vi "Build Report String.vi"(8 "error in (no error)":errorcluster, 10 "Result":T1, 11 "Timing Action in":refnum<class "Timing Action.lvclass">) -> (0 "error out":errorcluster, 2 "Report String":string, 3 "Timing Action out":refnum<class "Timing Action.lvclass">)   [LabVIEW 2020, in "MacroAssert.lvlib" / "Timing Action.lvclass"]
doc: "Builds a string using <B>Step</B> and <B>Result</B> to be included in a report."
uses:
  Timing Action.lvclass
  Timing Action.lvclass/Timing Action.ctl
  MacroAssert.lvlib
  Action Step/Action Step.lvclass
  CTLs/Result.ctl
  CTLs/Outcome.ctl
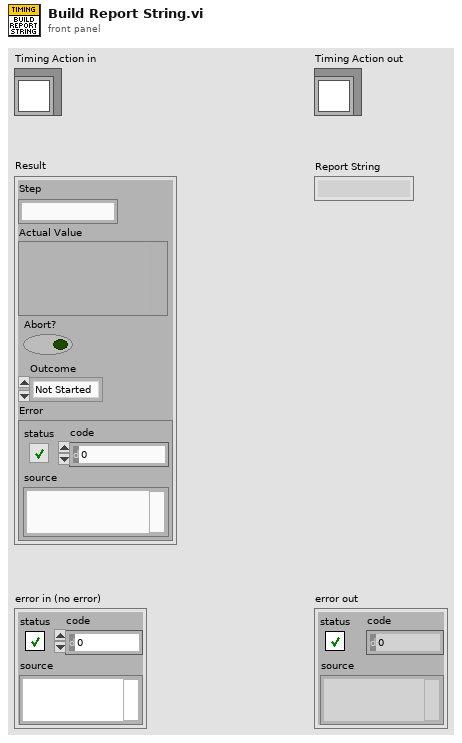
[diagram p1: front panel]
types:
  T1 = typedef "MacroAssert.lvlib/Result.ctl" = cluster{"Step":string, "Actual Value":variant, "Abort?":bool, "Outcome":T2, "Error":errorcluster}
  T2 = typedef "MacroAssert.lvlib/Outcome.ctl" = enum16{"Not Started", "Skipped", "Pass", "Fail", "Complete", "Error", "Auto Abort", "User Abort"}
  T3 = typedef "MacroAssert.lvlib/Timing Action.lvclass/Timing Action Type.ctl" = enum16{"Wait", "Wait Until"}
  T4 = typedef "MacroAssert.lvlib/Timing Action.lvclass/Time Unit.ctl" = enum16{"milliseconds", "seconds", "minutes"}
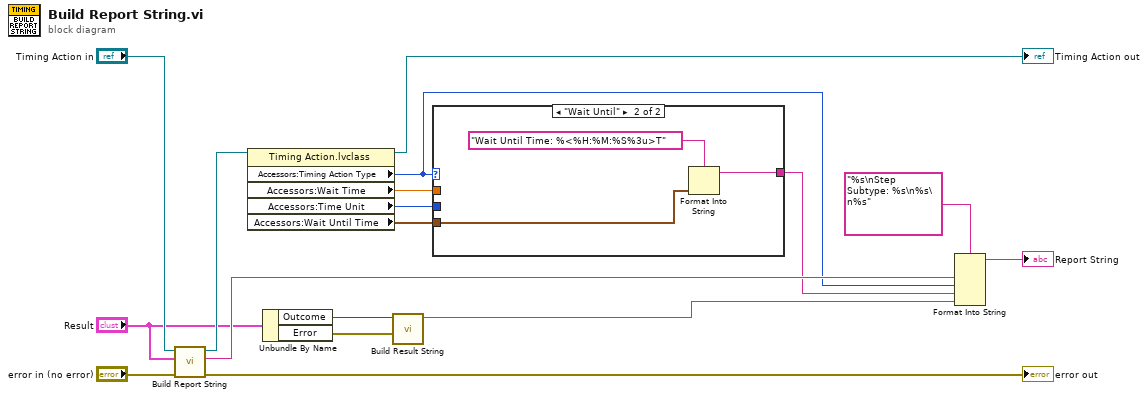
[diagram p0: block diagram]
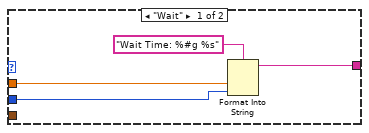
[diagram p2: hidden frame]
diagram:
  n1 = call-parent "Build Report String.vi"("error in (no error)"="error in (no error)", "Result"="Result", "Step in"="Timing Action in") -> ("error out"=→"error out":errorcluster, "Report String"=w12:string, "Step out"=w13:refnum<class "Timing Action.lvclass">)  [unwired: 6 in]
  n2 = property class="Timing Action.lvclass"(reference=w13) -> (reference out=→"Timing Action out":refnum<class "Timing Action.lvclass">, "Accessors:Timing Action Type"=w1:T3, "Accessors:Wait Time"=w5:dbl, "Accessors:Time Unit"=w4:T4, "Accessors:Wait Until Time"=w3:timestamp)  [unwired: 1 in, 1 out]
  n3 = Unbundle By Name("Result") -> ("Outcome"=w15:T2, "Error"=w17:errorcluster)
  n4 = call "Build Result String.vi"("Error"=w17, "Outcome"=w15) -> ("Result String"=w14:string)  [unwired: 9 in]
  n5 = case shown="\"Wait Until\"" w1 {
    tunnel: w5 -> [w20 _]
    tunnel: w4 -> [w19 _]
    tunnel: w3 -> [_ w23]
    tunnel: [w18 w22] -> w2
    frame "Wait" {
      n6 = Format Into String(format string="Wait Time: %#g %s", w20, w19) -> (resulting string=w18:string)  [unwired: 2 in, 1 out]
    }
    frame "Wait Until" {
      n7 = Format Into String(format string="Wait Until Time: %<%H:%M:%S%3u>T", w23) -> (resulting string=w22:string)  [unwired: 2 in, 1 out]
    }
  }
  n8 = Format Into String(format string="%s\nStep Subtype: %s\n%s\n%s", w12, w1, w2, w14) -> (resulting string=→"Report String":string)  [unwired: 2 in, 1 out]
